vi "图像对称、曲面操作.vi"() -> ()   [LabVIEW 2018]
uses:
  <vilib>/vision/NI_Vision_Development_Module.lvlib
panel:
  out "error out":errorcluster
  out "Image 2":T1(plugin-control)
  out "Image":T1(plugin-control)
  in  "路径":path
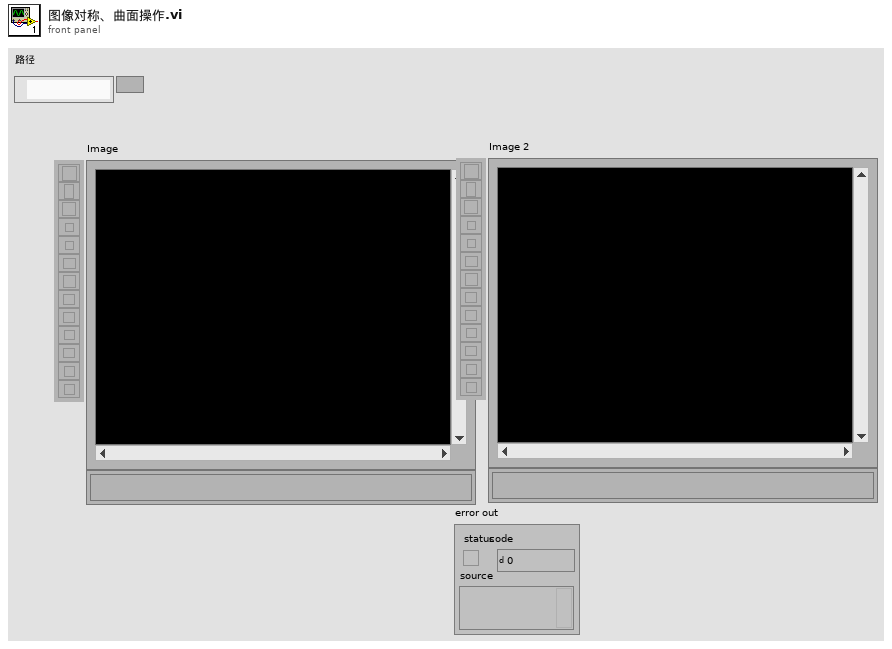
[diagram p1: front panel]
types:
  T1 = typedef "IMAQ Image.ctl" = refnum<image>
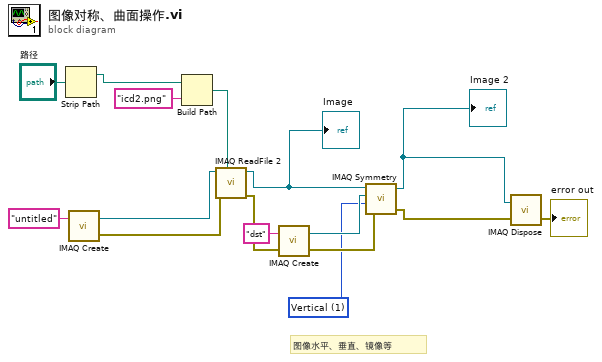
[diagram p0: block diagram]
diagram:
  w6 = u32 1 items=["Horizontal", "Vertical", "Central", "1st Diagonal", "2nd Diagonal"] ("Type of Symmetry")
  # "图像水平、垂直、镜像等"
  n1 = Strip Path(path="路径") -> (stripped path=w15:path)  [unwired: 1 out]
  n2 = call "IMAQ Create"("Image Name"="untitled") -> ("New Image"=w13:T1, "error out"=w12:errorcluster)  [unwired: 4 in]
  n3 = Build Path(base path=w15, name or relative path="icd2.png" ("名称或相对路径")) -> (appended path=w2:path)
  n4 = call "IMAQ ReadFile 2"("File Path"=w2, "error in (no error)"=w12, "Image"=w13) -> ("error out"=w10:errorcluster, "Image Out"=w5:T1)  [unwired: 4 in, 3 out]
  "Image" <- w5
  n5 = call "IMAQ Create"("Image Name"="dst", "error in (no error)"=w10) -> ("New Image"=w8:T1, "error out"=w7:errorcluster)  [unwired: 3 in]
  n6 = call "IMAQ Symmetry"("error in (no error)"=w7, "Type of Symmetry"=w6, "Image Dst"=w8, "Image Src"=w5) -> ("error out"=w3:errorcluster, "Image Dst Out"=w4:T1)  [unwired: 1 in]
  "Image 2" <- w4
  n7 = call "IMAQ Dispose"("Image"=w4, "error in (no error)"=w3) -> ("error out"=→"error out":errorcluster)  [unwired: 4 in]
